vi "GET_V_F.vi"(8 "error in (no error)":errorcluster caption="错误输入（无错误）", 11 "configuration file path":path caption="配置文件的路径") -> (0 "error out":errorcluster caption="错误输出", 2 "Version 2":string, 3 "FixtureNumber":string)   [LabVIEW 2018]
uses:
  <vilib>/Utility/config.llb/Read Key (String).vi
  <vilib>/Utility/config.llb/NI_LVConfig.lvlib
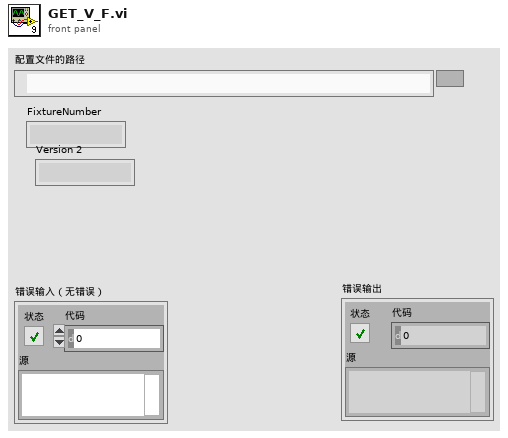
[diagram p1: front panel]
types:
  T1 = typedef "NI_LVConfig.lvlib/Config Data RefNum.ctl" = refnum<k1>
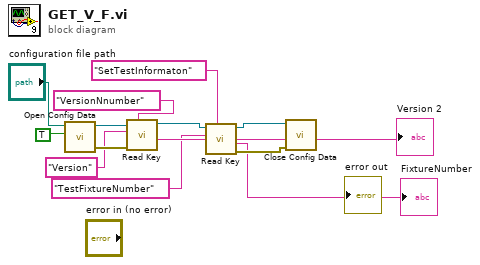
[diagram p0: block diagram]
diagram:
  n1 = call <vilib>:"Open Config Data.vi"("create file if necessary (T)"=TRUE, "configuration file path"="configuration file path") -> ("error out"=w8:errorcluster, "refnum"=w7:T1)  [unwired: 7 in, 1 out]
  n2 = call-poly <vilib>:"Read Key.vi"("section"="VersionNnumber", "error in (no error)"=w8, "key"="Version", "refnum"=w7) -> ("value"=→"Version 2":string, "refnum out"=w10:T1)  [unwired: 4 in, 2 out]
  n3 = call-poly <vilib>:"Read Key.vi"("section"="SetTestInformaton", "key"="TestFixtureNumber", "refnum"=w10) -> ("error out"=w13:errorcluster, "value"=→"FixtureNumber":string, "refnum out"=w12:T1)  [unwired: 5 in, 1 out]
  n4 = call <vilib>:"Close Config Data.vi"("error in (no error)"=w13, "refnum"=w12) -> ()  [unwired: 8 in, 2 out]
